vi "NIST myRIO time update.vi"(4 "error in (no error)":errorcluster, 6 "Session REF input":refnum<k21>="NI-myRIO-1900-03087726 (172.22.11.2)", 7 "Time Server IP Address (129.6.15.29)":string="129.6.15.29") -> (0 "error out":errorcluster)   [LabVIEW 2015]
uses:
  <vilib>/Utility/miscctls.llb/LVDateTimeRec.ctl
  <vilib>/nisyscfg/nisyscfg.lvlib
panel:
  out "time stamp":timestamp
  out "data out":string
  in  "Time Zone":string="CST"
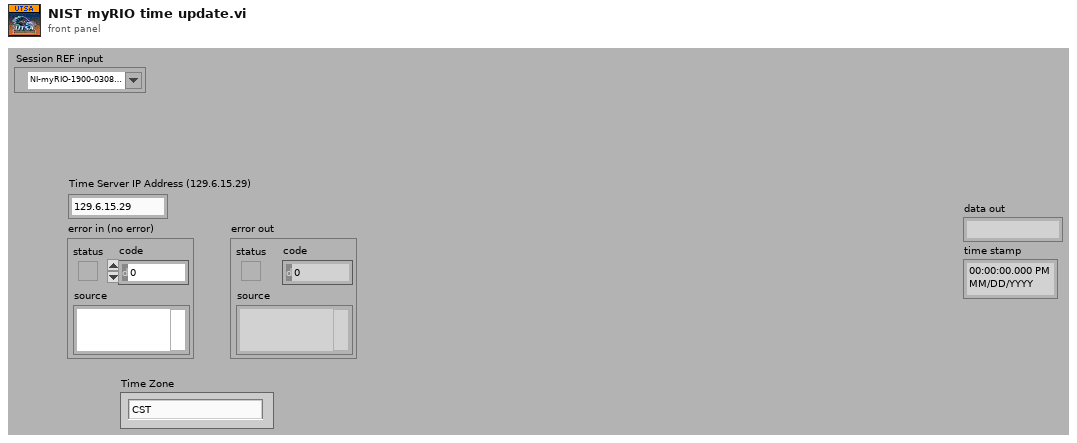
[diagram p1: front panel]
types:
  T1 = typedef "LVDateTimeRec.ctl" = cluster{"fractional second":dbl, "second":i32, "minute":i32, "hour":i32, "day of month":i32, "month":i32, "year":i32, "day of week":i32, "day of year":i32, "DST":i32}
  T2 = enum16{"Standard", "Buffered", "CRLF", "Immediate"}
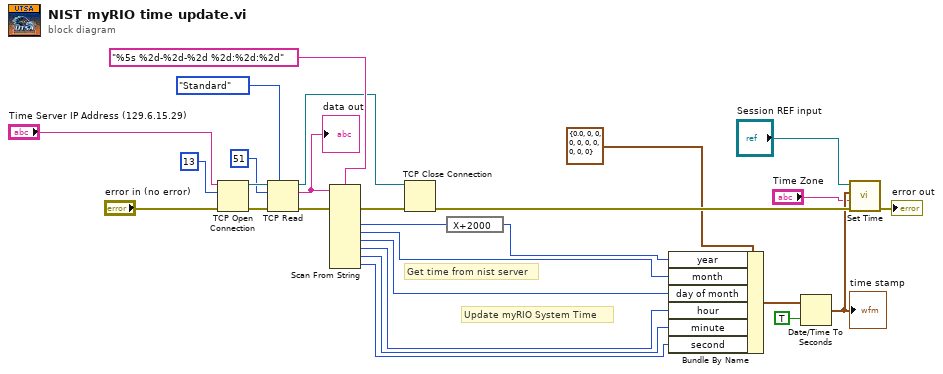
[diagram p0: block diagram]
diagram:
  # "Update myRIO System Time"
  # "Get time from nist server"
  n1 = TCP Open Connection(address="Time Server IP Address (129.6.15.29)", remote port or service name=u16 13 ("port"), error in (no error)="error in (no error)") -> (connection ID=w22:refnum<k5>, error out=w23:errorcluster)  [unwired: 2 in]
  n2 = TCP Read(connection ID=w22, bytes to read=51, error in (no error)=w23, 7:T2."Standard" ("mode (standard)")) -> (connection ID out=w16:refnum<k5>, data out=w8:string, error out=w19:errorcluster)  [unwired: 1 in]
  "data out" <- w8
  n3 = Scan From String(format string="%5s %2d-%2d-%2d %2d:%2d:%2d", input string=w8, error in=w19) -> (error out=w17:errorcluster, output 2=w26:i32, output 3=w10:i32, output 4=w11:i32, output 5=w12:i32, output 6=w13:i32, output 7=w14:i32)  [unwired: 9 in, 2 out]
  n4 = TCP Close Connection(connection ID=w16, error in (no error)=w17) -> (error out=w6:errorcluster)  [unwired: 1 in, 1 out]
  n5 = expression code="X+2000"(w26) -> (w9:i32)
  n6 = Bundle By Name(cluster=T1 {"fractional second"=0.0, "second"=0, "minute"=0, "hour"=0, "day of month"=0, "month"=0, "year"=0, "day of week"=0, "day of year"=0, "DST"=0} ("date time rec"), "year"=w9, "month"=w10, "day of month"=w11, "hour"=w12, "minute"=w13, "second"=w14) -> (w1:T1)
  n7 = Date/Time To Seconds(1:TRUE ("is UTC (F)"), 2:w1) -> (0:w4:timestamp)
  "time stamp" <- w4
  n8 = call <vilib>:"Set Time.vi"("error in (no error)"=w6, "Time Zone"="Time Zone", "Time"=w4, "Session in (localhost)"="Session REF input") -> ("error out"=→"error out":errorcluster)  [unwired: 4 in, 3 out]
